vi "SplitString.vi"(1 "Delimeter":string=" ", 2 "Name":string) -> (0 "Array":string[](array[string]))   [LabVIEW 2014]
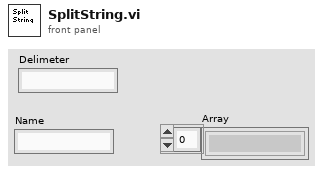
[diagram p1: front panel]
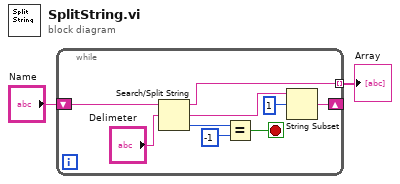
[diagram p0: block diagram]
diagram:
  n1 = while {
    tunnel: [w11] -> w1 mode=indexing
    shift-right: [w3] -> _
    shift-left: "Name" -> [w10]
    stop <- w6 stop-if-true
    n2 = Search/Split String(string=w10, search string/char (-)="Delimeter") -> (substring before match=w11:string, match + rest of string=w4:string, offset of match=w8:i32)  [unwired: 1 in]
    n3 = Equal?(x=w8, y=-1) -> (x = y?=w6:bool)
    n4 = String Subset(string=w4, offset (0)=1) -> (substring=w3:string)  [unwired: 1 in]
  }
  "Array" <- w1
